vi "FTW-Endpoint-Receive.vi"(0 "FTW Endpoint":refnum<class "FTW-Endpoint.lvclass">, 5 "Timeout":i32 format="%dmsec", 11 "error in":errorcluster) -> (4 "FTW Endpoint out":refnum<class "FTW-Endpoint.lvclass">, 6 "Message Header":string, 8 "Message Body":string, 10 "Timed out?":bool, 15 "error out":errorcluster)   [LabVIEW 2013, in "FTW-Endpoint.lvclass"]
uses:
  FTW-Endpoint.lvclass
  FTW-Endpoint.lvclass/FTW-Endpoint.ctl
panel:
  # "Inputs"
  # "Outputs"
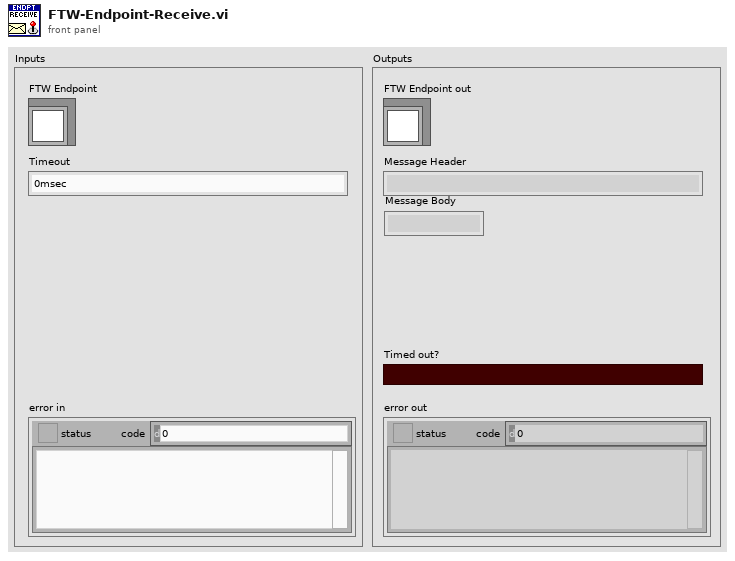
[diagram p1: front panel]
types:
  T1 = typedef "FTW-MessagePayload.ctl" = cluster{"Header":string, "Body":string, "Metadata":string}
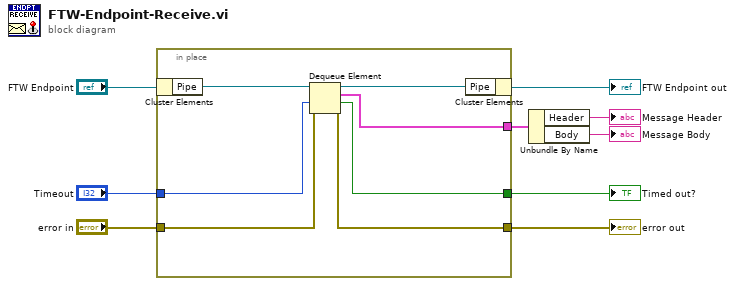
[diagram p0: block diagram]
diagram:
  n1 = in-place {
    in-place-border: [w13] -> w9
    in-place-border: "error in" -> [w14]
    in-place-border: "Timeout" -> [w15]
    in-place-border: [w11] -> w3
    in-place-border: [w10] -> w5
    n2 = in-place-cluster #1("FTW Endpoint") -> ("Pipe"=w16:refnum<queue>)
    n3 = Dequeue Element(queue=w16, timeout in ms (-1)=w15, error in (no error)=w14) -> (queue out=w12:refnum<queue>, element=w11:T1, timed out?=w10:bool, error out=w13:errorcluster)
    n4 = in-place-cluster #1("Pipe"=w12) -> (→"FTW Endpoint out":refnum<class "FTW-Endpoint.lvclass">)
  }
  "error out" <- w9
  "Timed out?" <- w5
  n5 = Unbundle By Name(w3) -> ("Header"=→"Message Header":string, "Body"=→"Message Body":string)
